vi "ExitRegUserEvent.vi"() -> (3 "ExitEvent":refnum<user-event>)   [LabVIEW 2024, in "Application.lvclass"]
uses:
  Application.lvclass
  Application.lvclass/Application.ctl
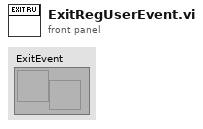
[diagram p1: front panel]
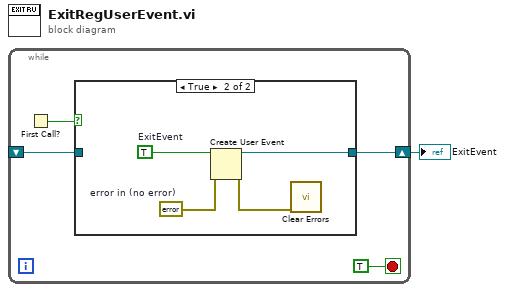
[diagram p0: block diagram]
diagram:
  n1 = while {
    shift-right: [w5] -> w1
    shift-left: _ -> [w3]
    stop <- TRUE stop-if-true
    n2 = First Call?() -> (First Call?: T/F=w4:bool)
    n3 = case shown="True" w4 {
      tunnel: [w6 w9] -> w5
      tunnel: w3 -> [w6 _]
      frame False {
      }
      frame True {
        w8 = errorcluster {"status"=FALSE, "code"=0, "source"=""}  # error in (no error)
        w10 = TRUE  # ExitEvent
        n4 = Create User Event(user event datatype=w10, error in=w8) -> (user event=w9:refnum<user-event>, error out=w7:errorcluster)
        n5 = call <vilib>:"Clear Errors.vi"("error in (no error)"=w7) -> ()  [unwired: 5 in, 2 out]
      }
    }
  }
  "ExitEvent" <- w1
